vi "Set Relays.vi"(8 "error in":errorcluster, 10 "Channel numbers":u8[](array[numeric]), 11 "task in":i32) -> (0 "error out":errorcluster, 3 "task out":i32)   [LabVIEW 2023, in "DO_Relay.lvlib"]
uses:
  <userlib>/DAQNavi Polymorphic VI/write/DAQNavi Write (Digtial 1D U8 NChan 1Samp).vi
  DO_Relay.lvlib
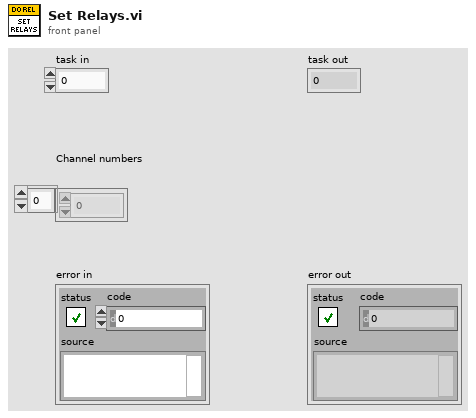
[diagram p1: front panel]
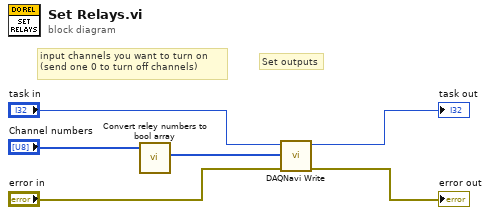
[diagram p0: block diagram]
diagram:
  # "Set outputs"
  # "input channels you want to turn on\n(send one 0 to turn off channels)"
  n1 = call "Convert reley numbers to bool array.vi"("Channels  numbers"="Channel numbers") -> ("Channels converted"=w5:u8[])  [unwired: 9 in, 1 out]
  n2 = call-poly <userlib>:"DAQNavi Write.vi"("error in (no error)"="error in", "data"=w5, "task in"="task in") -> ("error out"=→"error out":errorcluster, "task out"=→"task out":i32)  [unwired: 1 in, 6 out]
